vi "find serial port.vi"(0 "target version":dbl=1.0, 5 "error in (no error)":errorcluster) -> (14 "VISA resource name out":refnum<visa-resource-name>, 15 "port opened":bool, 16 "version":dbl, 17 "message":string, 18 "version too high":bool, 19 "error out":errorcluster)   [LabVIEW 2017]
uses:
  <vilib>/Instr/_visa.llb/VISA Find Search Mode.ctl
panel:
  out "all versions":dbl[](array[numeric])
  out "all openable ports":refnum<visa-resource-name>[](array[refnum])
  out "all messages":string[](array[string])
  out "find list":string[](array[string])
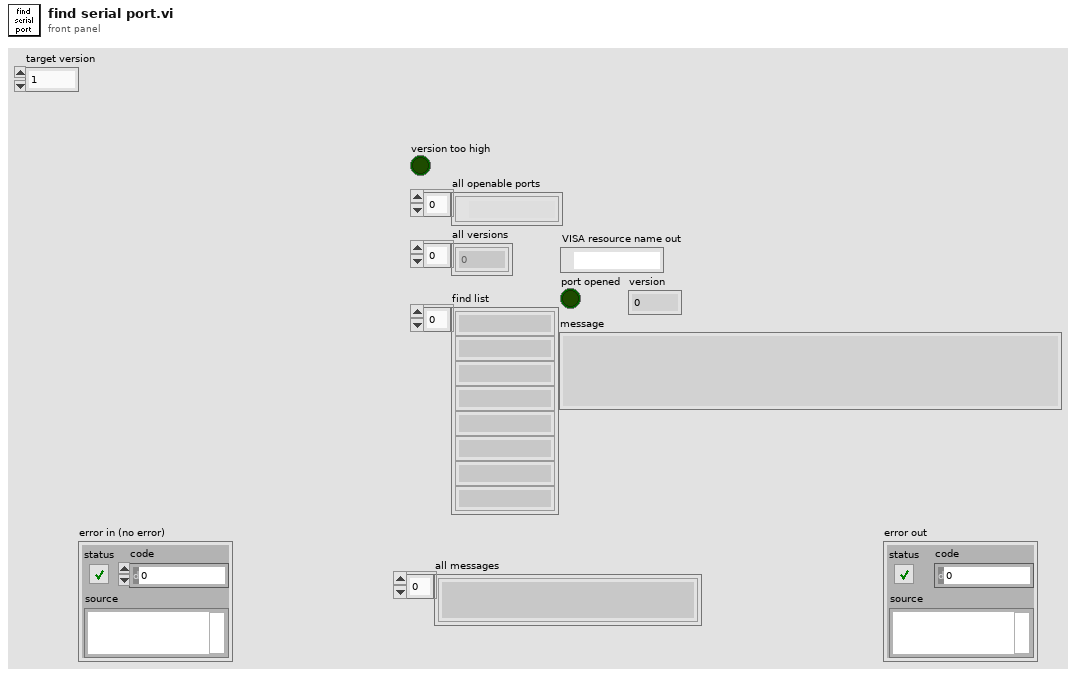
[diagram p1: front panel]
types:
  T1 = typedef "VISA Find Search Mode.ctl" = u32
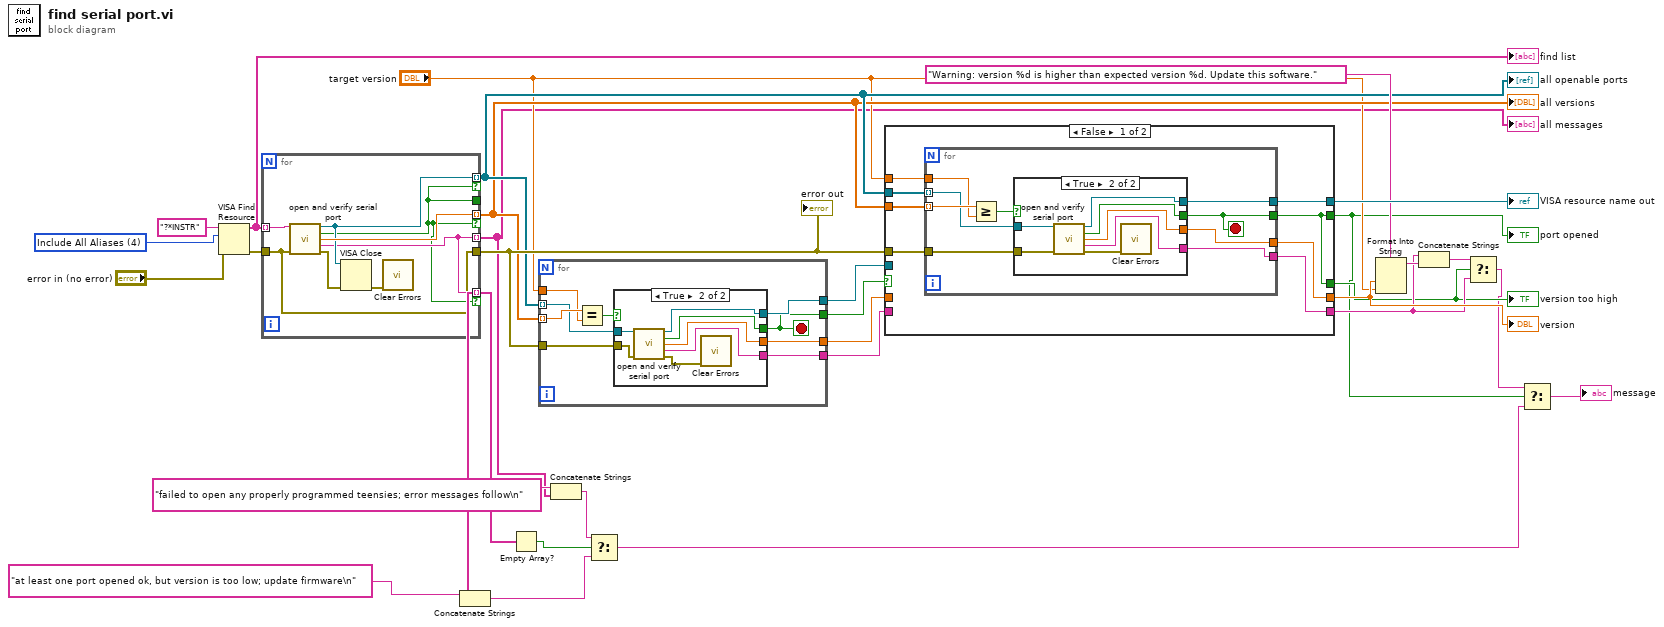
[diagram p0: block diagram]
diagram:
  w30 = T1 4 items=["Canonical Names Only"=0, "Aliases Only"=2, "Include Matching Aliases"=3, "Include All Aliases"=4] ("Search Mode")
  n1 = VISA Find Resource(8:"error in (no error)", 10:w30, 11:"?*INSTR" ("expression (\"?*\")")) -> (0:w29:errorcluster, 3:w28:string[])  [unwired: 1 out]
  "find list" <- w28
  n2 = for {
    tunnel: w29 -> [w32]
    tunnel: w28 -> [w39] mode=indexing
    tunnel: [w36] -> w15 mode=indexing if=w33
    tunnel: [w34] -> w7 mode=indexing
    tunnel: [w33] -> _
    tunnel: [w38] -> w14 mode=indexing if=w33
    tunnel: [w32] -> w26
    tunnel: [w34] -> w12 mode=indexing if=w33
    n3 = call "open and verify serial port.vi"("VISA resource name"=w39, "error in (no error)"=w32) -> ("VISA resource name out"=w36:refnum<visa-resource-name>, "port opened"=w33:bool, "version"=w38:dbl, "message"=w34:string, "error out"=w37:errorcluster)  [unwired: 9 in]
    n4 = VISA Close(VISA resource name=w36, error in (no error)=w37) -> (error out=w35:errorcluster)
    n5 = call <vilib>:"Clear Errors.vi"("error in (no error)"=w35) -> ()  [unwired: 5 in, 2 out]
  }
  "all messages" <- w7
  "all openable ports" <- w15
  "all versions" <- w14
  "error out" <- w26
  n6 = Concatenate Strings("at least one port opened ok, but version is too low; update firmware\n", w12) -> (w9:string)
  n7 = Empty Array?(array=w12) -> (empty?=w11:bool)
  n8 = for {
    tunnel: w14 -> [w48] mode=indexing
    tunnel: w15 -> [w46] mode=indexing
    tunnel: w26 -> [w45]
    tunnel: [w44] -> w25
    tunnel: [w43] -> w24
    tunnel: [w42] -> w23
    tunnel: [w41] -> w27
    tunnel: "target version" -> [w40]
    stop <- w41 stop-if-true
    n9 = Equal?(x=w48, y=w40) -> (x = y?=w47:bool)
    n10 = case shown="True" w47 {
      tunnel: w46 -> [_ w55]
      tunnel: w45 -> [_ w54]
      tunnel: [_ w53] -> w44
      tunnel: [_ w52] -> w41
      tunnel: [_ w51] -> w43
      tunnel: [_ w50] -> w42
      frame False {
      }
      frame True {
        n11 = call "open and verify serial port.vi"("VISA resource name"=w55, "error in (no error)"=w54) -> ("VISA resource name out"=w53:refnum<visa-resource-name>, "port opened"=w52:bool, "version"=w51:dbl, "message"=w50:string, "error out"=w49:errorcluster)  [unwired: 9 in]
        n12 = call <vilib>:"Clear Errors.vi"("error in (no error)"=w49) -> ()  [unwired: 5 in, 2 out]
      }
    }
  }
  n13 = Concatenate Strings("failed to open any properly programmed teensies; error messages follow\n" ("string"), w7) -> (w6:string)
  n14 = Select(t=w6, s=w11, f=w9) -> (s? t:f=w3:string)
  n15 = case shown="False" w27 {
    selector: w27 -> [_ w80]
    tunnel: w15 -> [w63 _]
    tunnel: w14 -> [w62 _]
    tunnel: "target version" -> [w61 _]
    tunnel: w26 -> [w60 _]
    tunnel: w25 -> [_ w83]
    tunnel: w24 -> [_ w81]
    tunnel: w23 -> [_ w82]
    tunnel: [w59 w83] -> w22
    tunnel: [w58 w81] -> w20
    tunnel: [w57 w82] -> w17
    tunnel: [w56 w80] -> w4
    tunnel: [w56 _] -> w16
    frame False {
      n16 = for {
        tunnel: w62 -> [w72] mode=indexing
        tunnel: w63 -> [w70] mode=indexing
        tunnel: w60 -> [w69]
        tunnel: [w68] -> w59
        tunnel: [w67] -> w58
        tunnel: [w66] -> w57
        tunnel: [w65] -> w56
        tunnel: w61 -> [w64]
        stop <- w65 stop-if-true
        n17 = Greater Or Equal?(x=w72, y=w64) -> (x >= y?=w71:bool)
        n18 = case shown="True" w71 {
          tunnel: w70 -> [_ w79]
          tunnel: w69 -> [_ w78]
          tunnel: [_ w77] -> w68
          tunnel: [_ w76] -> w65
          tunnel: [_ w75] -> w67
          tunnel: [_ w74] -> w66
          frame False {
          }
          frame True {
            n19 = call "open and verify serial port.vi"("VISA resource name"=w79, "error in (no error)"=w78) -> ("VISA resource name out"=w77:refnum<visa-resource-name>, "port opened"=w76:bool, "version"=w75:dbl, "message"=w74:string, "error out"=w73:errorcluster)  [unwired: 9 in]
            n20 = call <vilib>:"Clear Errors.vi"("error in (no error)"=w73) -> ()  [unwired: 5 in, 2 out]
          }
        }
      }
    }
    frame True {
    }
  }
  "VISA resource name out" <- w22
  "port opened" <- w4
  "version" <- w20
  "version too high" <- w16
  n21 = Format Into String(format string="Warning: version %d is higher than expected version %d. Update this software.", w20, "target version") -> (resulting string=w19:string)  [unwired: 2 in, 1 out]
  n22 = Concatenate Strings(w17, w19) -> (w18:string)
  n23 = Select(t=w18, s=w16, f=w17) -> (s? t:f=w5:string)
  n24 = Select(t=w5, s=w4, f=w3) -> (s? t:f=→"message":string)
